vi "Predict Search Rectangle from Particle.vi"(8 "Margin":dbl[](array[numeric])=[-15.0, -15.0, 15.0, 15.0], 11 "Sorted Data":dbl[](array[numeric])) -> (0 "ROI Descriptor":T1 {"Contours"."Type" items=["No Selection", "Point", "Line", "Rectangle", "Oval", "Polygon", "Freehand Region", "Annulus", "Unused2", "Unused3", "Broken Line", "Freehand Line", "Rotated Rectangle"]}, 2 "Valid":bool, 3 "Rectangle ltrb":dbl[](array[numeric]))   [LabVIEW 2013]
doc: "Given the rectangle descriptor around the particle, calculate where to search for the ball. Produces a rectangle, an RIO, and whether the rectangle makes sense."
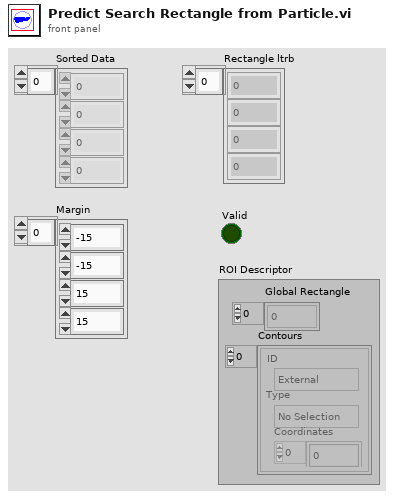
[diagram p1: front panel]
types:
  T1 = typedef "ROI Descriptor" = cluster{"Global Rectangle":i32[], "Contours":cluster{"ID":enum32{"External", "Internal"}, "Type":u32, "Coordinates":i32[]}[]}
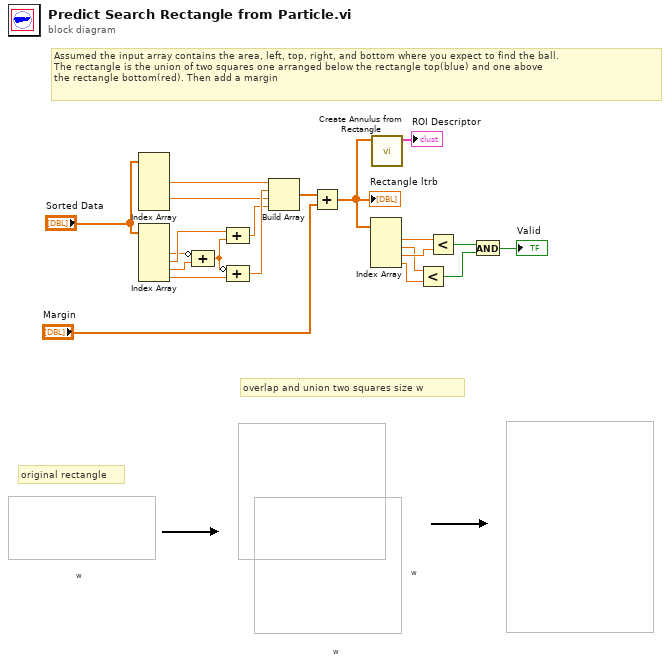
[diagram p0: block diagram]
diagram:
  # "overlap and union two squares size w"
  # "original rectangle"
  # "w"
  # "w"
  # "w"
  # "Assumed the input array contains the area, left, top, right, and bottom where you expect to find the ball.\nThe rectangle is the union of two squares one arranged below the rectangle top(blue) and one above\nthe rectangle bottom(red). Then add a margin"
  n1 = Index Array(array="Sorted Data") -> (element #2=w18:dbl, element #4=w17:dbl)  [unwired: 5 in, 3 out]
  n2 = Index Array(array="Sorted Data") -> (element #2=w11:dbl, element #3=w13:dbl, element #4=w12:dbl, element #5=w15:dbl)  [unwired: 5 in, 1 out]
  n3 = Compound Arithmetic op=ADD(invert w11, w12) -> (w14:dbl)
  n4 = Compound Arithmetic op=ADD(w13, w14) -> (w19:dbl)
  n5 = Compound Arithmetic op=ADD(invert w14, w15) -> (w20:dbl)
  n6 = Build Array(w18, w20, w17, w19) -> (w21:dbl[])
  n7 = Add(x=w21, y="Margin") -> (x+y=w2:dbl[])
  "Rectangle ltrb" <- w2
  n8 = Index Array(array=w2) -> (element #1=w9:dbl, element #2=w7:dbl, element #3=w8:dbl, element #4=w6:dbl)  [unwired: 4 in]
  n9 = call "Create Annulus from Rectangle.vi"("Rectangle ltrb"=w2) -> ("ROI Descriptor"=→"ROI Descriptor":T1)  [unwired: 10 in]
  n10 = Less?(x=w7, y=w6) -> (x < y?=w4:bool)
  n11 = Less?(x=w9, y=w8) -> (x < y?=w5:bool)
  n12 = And(x=w5, y=w4) -> (x .and. y?=→"Valid":bool)
